vi "loadingbar.vi"(8 "error in":errorcluster) -> (0 "error out":errorcluster)   [LabVIEW 2019]
uses:
  <vilib>/Utility/miscctls.llb/LVPointTypeDef.ctl
  Load Glb.vi
  Commonly VI.lvlib
panel:
  in  "Tab Control":enum32{"Page 1"}(tab)
  out "Horizontal Graduated Bar":i32(slide) caption="DataLoading....." scale=0.0..100.0
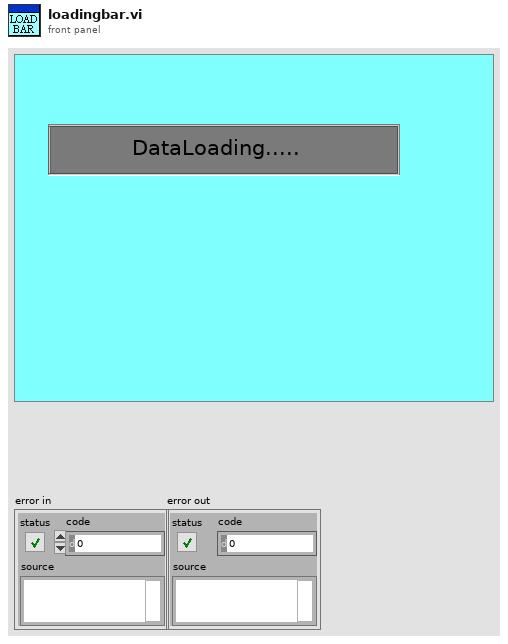
[diagram p1: front panel]
types:
  T1 = typedef "LVPointTypeDef.ctl" = cluster{"Horizontal":i16, "Vertical":i16}
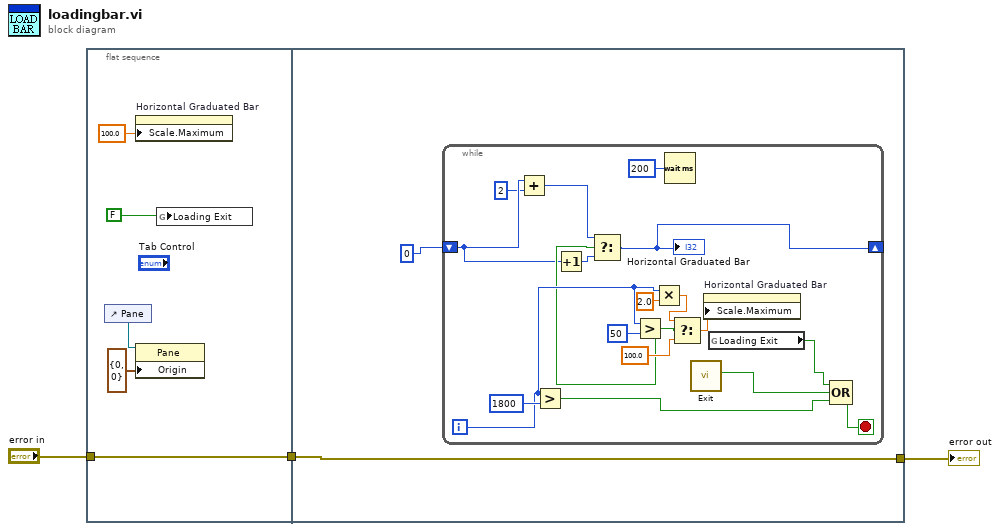
[diagram p0: block diagram]
diagram:
  n1 = flat-sequence {
    tunnel: [w8] -> w3
    tunnel: "error in" -> [w8]
    tunnel: [w10] -> w1
    tunnel: w3 -> [w10]
    frame #0 {
      n2 = control-ref of="Pane"() -> (w7:refnum<vi>)
      n3 = property on="Horizontal Graduated Bar" class="Slide (strict)"("Scale.Maximum"=100.0 ("Scale.Range:Maximum")) -> ()  [unwired: 2 in, 2 out]
      n4 = property class="Pane"(reference=w7, "Origin"=T1 {"Horizontal"=0, "Vertical"=0}) -> ()  [unwired: 1 in, 2 out]
      n5 = global write "Load Glb.vi" "Loading Exit"(FALSE ("LoadingExit")) -> ()
    }
    frame #1 {
      n6 = while {
        shift-right: [w16] -> _
        shift-left: 0 ("Horizontal Graduated Bar") -> [w14]
        i -> [w18]
        stop <- w27 stop-if-true
        n7 = Add(x=w14, y=2) -> (x+y=w13:i32)
        n8 = Greater?(x=w18, y=1800) -> (0:w26:bool)
        n9 = Increment(x=w14) -> (x+1=w17:i32)
        n10 = Greater?(x=w18, y=50) -> (0:w15:bool)
        n11 = Select(t=w13, s=w15, f=w17) -> (s? t:f=w16:i32)
        "Horizontal Graduated Bar" <- w16
        n12 = Multiply(x=w18, y=2.0) -> (x*y=w20:dbl)
        n13 = Wait (ms)(milliseconds to wait=u32 200) -> ()  [unwired: 1 out]
        n14 = Select(t=w20, s=w15, f=100.0) -> (s? t:f=w21:dbl)
        n15 = call "Exit.vi"() -> ("ExitOut"=w25:bool)  [unwired: 11 in]
        n16 = property on="Horizontal Graduated Bar" class="Slide (strict)"("Scale.Maximum"=w21) -> ()  [unwired: 2 in, 2 out]
        n17 = global read "Load Glb.vi" "Loading Exit"() -> (w11:bool)
        n18 = Compound Arithmetic op=OR(w11, w25, w26) -> (w27:bool)
      }
    }
  }
  "error out" <- w1
